vi "Transform.vi"(7 "Type X":T2(ring), 8 "error in (no error)":errorcluster caption="entrée d'erreur (pas d'erreur)", 9 "y":string[][](array[string]), 10 "X":string[][](array[string]), 11 "RBFSampler.lvclass":refnum<class "RBFSampler.lvclass">) -> (0 "error out":errorcluster caption="sortie d'erreur", 2 "Data":T1, 3 "RBFSampler.lvclass":refnum<class "RBFSampler.lvclass">)   [LabVIEW 2020, in "RBFSampler.lvclass"]
doc: "Apply the approximate feature map to X.\n\nReturns : \n\n- X_new : array-like, shape (n_samples, n_components)"
uses:
  RBFSampler.lvclass
  RBFSampler.lvclass/RBFSampler.ctl
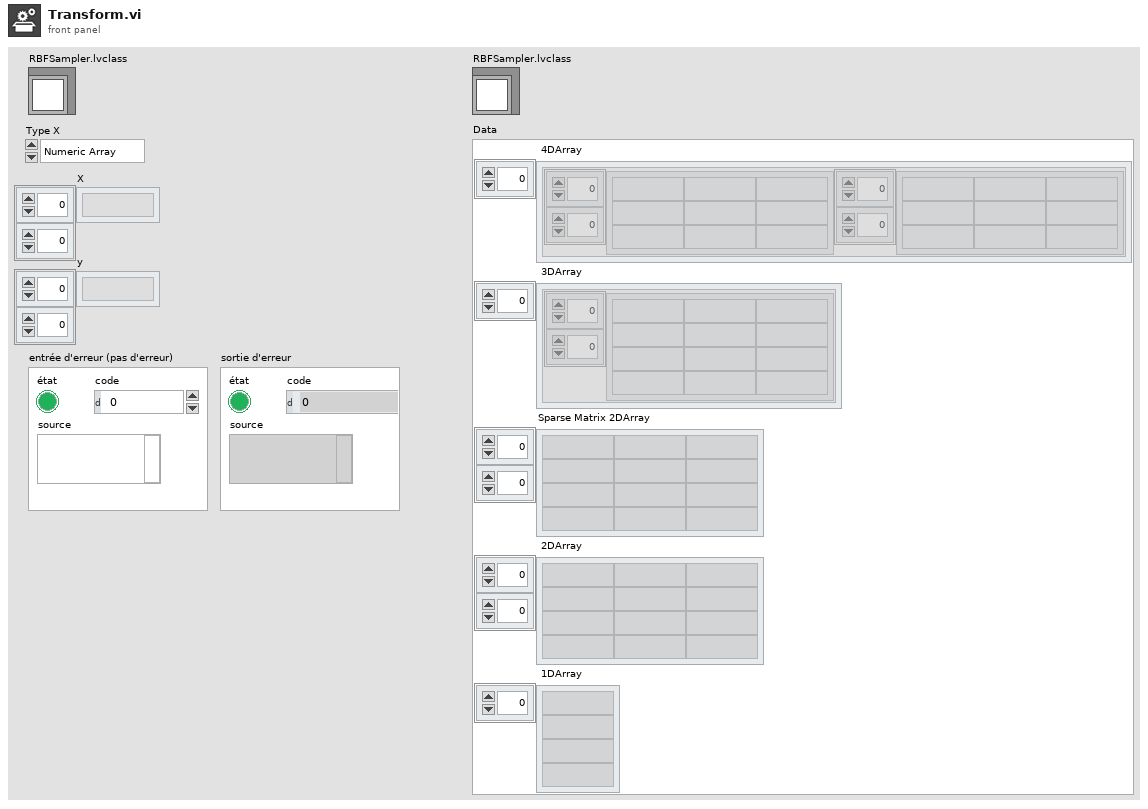
[diagram p1: front panel]
types:
  T1 = cluster{" 4DArray":cluster{"1":string[][], "2":string[][]}[], " 3DArray":cluster{"Tableau":string[][]}[], "Sparse Matrix 2DArray":string[][], " 2DArray":string[][], " 1DArray":string[]}
  T2 = enum16{"Numeric Array", "String Array", "Sparse"}
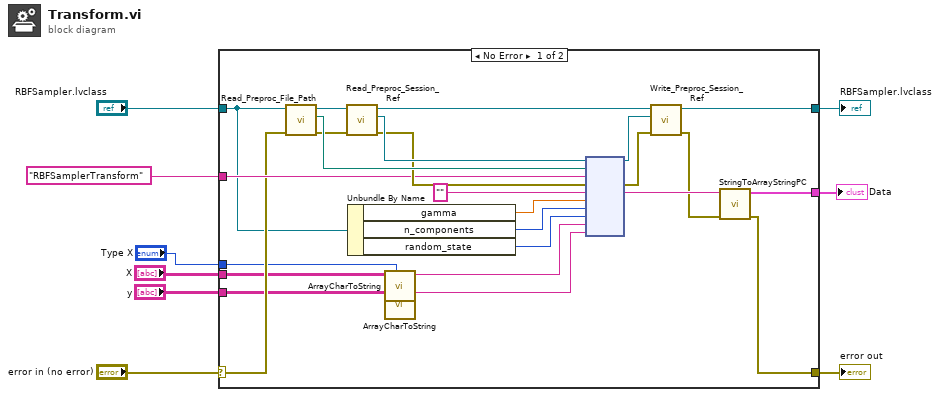
[diagram p0: block diagram]
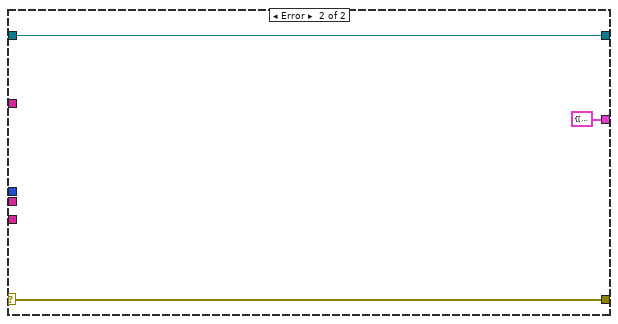
[diagram p2: hidden frame]
diagram:
  n1 = case shown="No Error" "error in (no error)" {
    selector: "error in (no error)" -> [w22 w37]
    tunnel: [w11 w37] -> w8
    tunnel: [w19 w36] -> w6
    tunnel: "RBFSampler.lvclass" -> [w21 w36]
    tunnel: "RBFSamplerTransform" ("Fonction") -> [w23 _]
    tunnel: "X" -> [w18 _]
    tunnel: "y" -> [w16 _]
    tunnel: "Type X" -> [w17 _]
    tunnel: [w10 T1 {" 4DArray"=[], " 3DArray"=[], "Sparse Matrix 2DArray"=[], " 2DArray"=[], " 1DArray"=[]} ("Data")] -> w1
    frame No Error {
      n2 = call-dynamic "Read_Preproc_File_Path.vi"("error in (no error)"=w22, "Python in"=w21) -> ("error out"=w29:errorcluster, "File_Path"=w32:path, "Python out"=w34:refnum<class "RBFSampler.lvclass">)  [unwired: 7 in]
      n3 = call-dynamic "Read_Preproc_Session_Ref.vi"("error in (no error)"=w29, "Python in"=w34) -> ("error out"=w30:errorcluster, "Session_ref"=w31:refnum<k35>, "Python out"=w33:refnum<class "RBFSampler.lvclass">)  [unwired: 7 in]
      n4 = Unbundle By Name(w21) -> ("gamma"=w25:dbl, "n_components"=w24:i32, "random_state"=w20:i32)
      n5 = call "ArrayCharToString.vi"("Type"=w17, "TAB"=w18) -> ("Instruction"=w15:string)  [unwired: 9 in]
      n6 = call "ArrayCharToString.vi"("TAB"=w16) -> ("Instruction"=w14:string)  [unwired: 10 in]
      n7 = node(w31, w32, w23, w30, "", w25, w24, w20, w15, w14) -> (w26:refnum<k35>, w28:errorcluster, w13:string)  [unwired: 5 in, 2 out]
      n8 = call-dynamic "Write_Preproc_Session_Ref.vi"("error in (no error)"=w28, "Session_ref"=w26, "Python in"=w33) -> ("error out"=w12:errorcluster, "Python out"=w19:refnum<class "RBFSampler.lvclass">)  [unwired: 7 in]
      n9 = call "StringToArrayStringPC.vi"("sortie d'erreur"=w12, "Return value"=w13) -> ("sortie d'erreur"=w11:errorcluster, "Data"=w10:T1)  [unwired: 8 in]
    }
    frame Error {
    }
  }
  "error out" <- w8
  "RBFSampler.lvclass" <- w6
  "Data" <- w1
